vi "Correct for MIO inter-channel delay (continuous).vi"() -> ()   [LabVIEW 2020]
doc: "When acquiring waveforms from channels of a data acquisition card that uses a single A/D with a multiplexer, the different channels will not be sampled at the same points in time. This example demonstrates the use of resampling and alignment to correct for this inter-channel delay, resulting in a simultaneously sampled set of waveforms."
uses:
  <vilib>/measure/maresamp.llb/Align N Waveforms (continuous).vi
  <vilib>/measure/matone.llb/Extract Single Tone Information N Chan.vi
  <vilib>/measure/NI_MAPro.lvlib
panel:
  in  "Stop":bool
  out "Max amplitude mismatch (%)":dbl format="%#.6g"
  out "Max phase mismatch (deg)":dbl
  out "Re-aligned Waveforms":waveform(dbl)[](graph)
  out "Input Waveforms":waveform(dbl)[](graph)
  # "Overview: Demonstrates the use of resampling and alignment to correct for the inter-channel delay in multiplexed data.\nRequirements: LabVIEW Full Development System\nInstructions:\n1. Run the VI. The Input Waveforms graph shows four channels of data, each sampled at different time offsets.  In the Re-aligned Waveforms graph, all the plots line up with no offset.\n2. Click Stop to stop the VI."
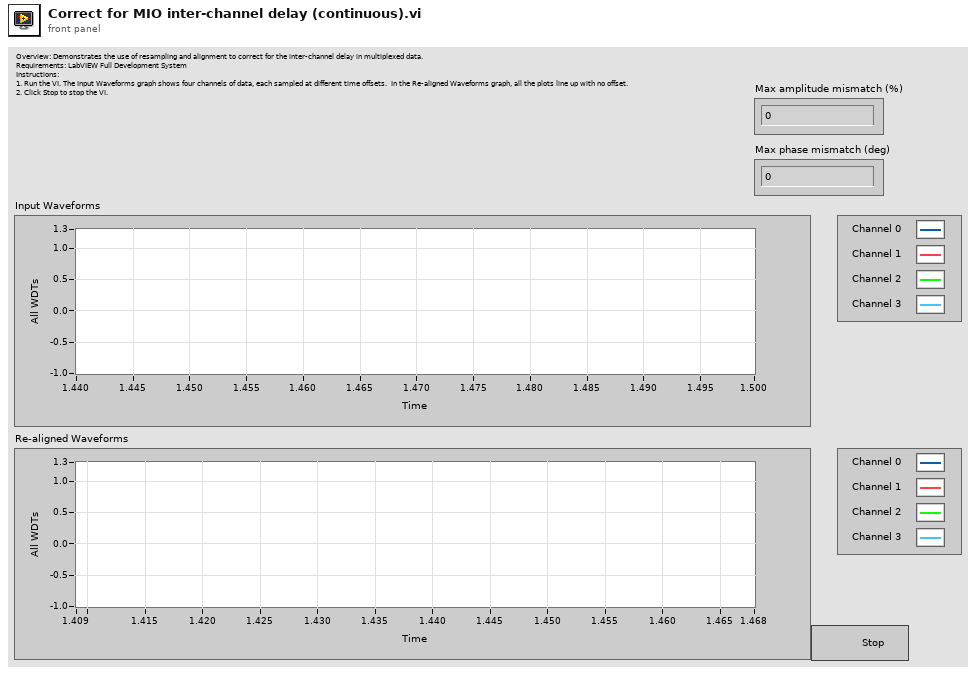
[diagram p1: front panel]
types:
  T1 = cluster{"alias rejection (dB)":dbl, "normalized bandwidth":dbl}
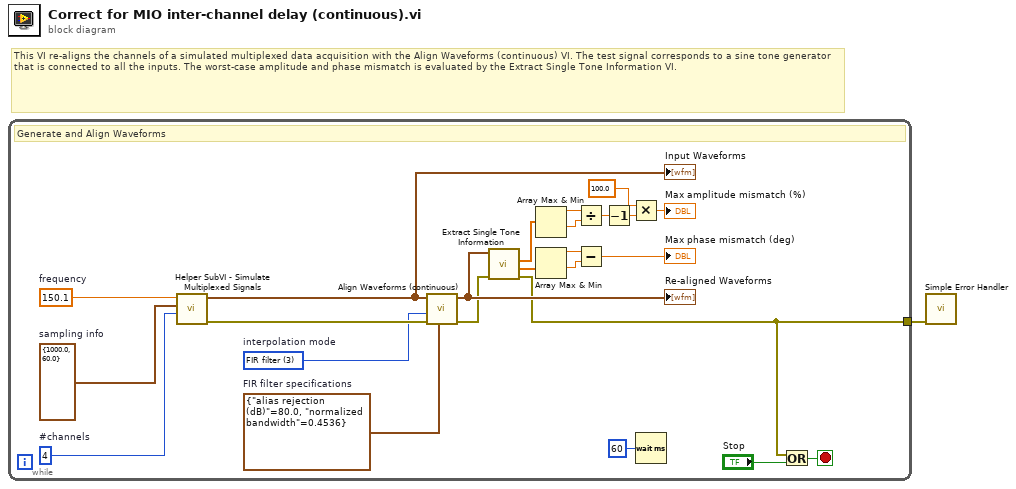
[diagram p0: block diagram]
diagram:
  # "This VI re-aligns the channels of a simulated multiplexed data acquisition with the Align Waveforms (continuous) VI. The test signal corresponds to a sine tone generator that is connected to all the inputs. The worst-case amplitude and phase mismatch is evaluated by the Extract Single Tone Information VI."
  n1 = while {
    tunnel: [w4] -> w1
    stop <- w5 stop-if-true
    w2 = 4  # #channels
    w3 = cluster{"Fs":dbl, "#s":dbl} {"Fs"=1000.0, "#s"=60.0}  # sampling info
    w22 = 150.1  # frequency
    w24 = T1 {"alias rejection (dB)"=80.0, "normalized bandwidth"=0.4536}  # FIR filter specifications
    w7 = u16 3 items=["coerce", "linear", "spline", "FIR filter"]  # interpolation mode
    # "Generate and Align Waveforms"
    n2 = call "Helper SubVI - Simulate Multiplexed Signals.vi"("#channels"=w2, "sampling info"=w3, "frequency"=w22) -> ("error out"=w23:errorcluster, "signal array out"=w17:waveform(dbl)[])  [unwired: 3 in, 4 out]
    "Input Waveforms" <- w17
    n3 = call-poly <vilib>:"Align Waveforms (continuous).vi"("FIR filter specifications"=w24, "error in (no error)"=w23, "interpolation mode"=w7, "waveforms in"=w17) -> ("error out"=w6:errorcluster, "waveforms out"=w16:waveform(dbl)[])  [unwired: 2 in, 4 out]
    "Re-aligned Waveforms" <- w16
    n4 = call-poly <vilib>:"Extract Single Tone Information.vi"("error in (no error)"=w6, "time signals in"=w16) -> ("error out"=w4:errorcluster, "detected phases (deg)"=w21:dbl[], "detected amplitudes"=w13:dbl[])  [unwired: 2 in, 5 out]
    n5 = Array Max & Min(array=w13) -> (max value=w14:dbl, min value=w15:dbl)  [unwired: 2 out]
    n6 = Array Max & Min(array=w21) -> (max value=w20:dbl, min value=w19:dbl)  [unwired: 2 out]
    n7 = Divide(x=w14, y=w15) -> (x/y=w12:dbl)
    n8 = Subtract(x=w20, y=w19) -> (x-y=→"Max phase mismatch (deg)":dbl)
    n9 = Decrement(x=w12) -> (x-1=w11:dbl)
    n10 = Multiply(x=100.0, y=w11) -> (x*y=→"Max amplitude mismatch (%)":dbl)
    n11 = Wait (ms)(milliseconds to wait=u32 60) -> ()  [unwired: 1 out]
    n12 = Or(x=w4, y="Stop") -> (x .or. y?=w5:bool)
  }
  n13 = call <vilib>:"Simple Error Handler.vi"("error in (no error)"=w1) -> ()  [unwired: 4 in, 5 out]
